vi "XY Graph Compute Sliced Mean & SDV Plots.vi"(8 "error in (no error)":errorcluster, 10 "Plot":cluster{"X Array":dbl[], "Y Array":dbl[]}, 11 "Slices Definition":T1={"Axis Start"=0.0, "Axis Stop"=0.0, "# Steps"=0, "Step Size"=1.0, "Step Definition"=enum."# Steps", "Upper Percentile"=1.0, "Lower Percentile"=1.0, "Min # Data Points/Slice"=1, "Output Abscissa Statistics Plots"=FALSE} {"Min # Data Points/Slice" min=0 max=100; "Lower Percentile" min=0.0 max=100.0; "Upper Percentile" min=0.0 max=100.0; "Step Size" min=1.0; "# Steps" min=1}) -> (0 "error out":errorcluster, 3 "Plots":cluster{"X Array":dbl[], "Y Array":dbl[]}[](array[cluster]))   [LabVIEW 2021, in "XY Graph Add-Ons.lvlib"]
uses:
  XY Graph Add-Ons.lvlib
  XY Graph Slides Mean & SDV Step Definition.ctl
  Arrays/Linear Ramp End Options.ctl
  49f03c9f-9bb8-4480-9460-08b8970c46f1.vi
  f2368cde-c411-4778-92ad-cdfa6392accb.vi
  ad4c9e8f-85ce-46f2-8889-cace00dc3fba.vi
  <userlib>/_OpenG.lib/array/array.llb/Sort 1D Array (DBL)__ogtk.vi
  <vilib>/Utility/error.llb/Error Cluster From Error Code.vi
  <vilib>/ErrorRing/Error Ring.xnode
  <vilib>/Comparison/Less/Less Functor/Less Functor.lvclass
  <vilib>/gmath/statdist.llb/st_Percentiles (array).vi
  <userlib>/_OpenG.lib/array/array.llb/Reorder 1D Array2 (DBL)__ogtk.vi
  Arrays/Arrays.lvlib
  <userlib>/_OpenG.lib/array/array.llb/openg_array.lvlib
  <vilib>/gmath/NI_Gmath.lvlib
  Comparison/Comparison.lvlib
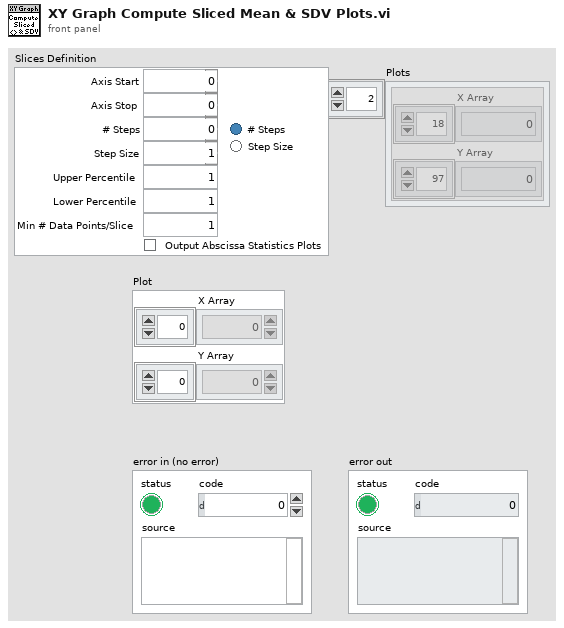
[diagram p1: front panel]
types:
  T1 = typedef "XY Graph Add-Ons.lvlib/XY Graph Slides Mean & SDV Step Definition.ctl" = cluster{"Axis Start":dbl, "Axis Stop":dbl, "# Steps":i32, "Step Size":dbl, "Step Definition":enum32{"# Steps", "Step Size"}, "Upper Percentile":dbl, "Lower Percentile":dbl, "Min # Data Points/Slice":i32, "Output Abscissa Statistics Plots":bool}
  T2 = typedef "Arrays.lvlib/Linear Ramp End Options.ctl" = enum16{"Include Min/Exclude Max", "Exclude Min/Include Max", "Include Both Ends", "Exclude Both Ends"}
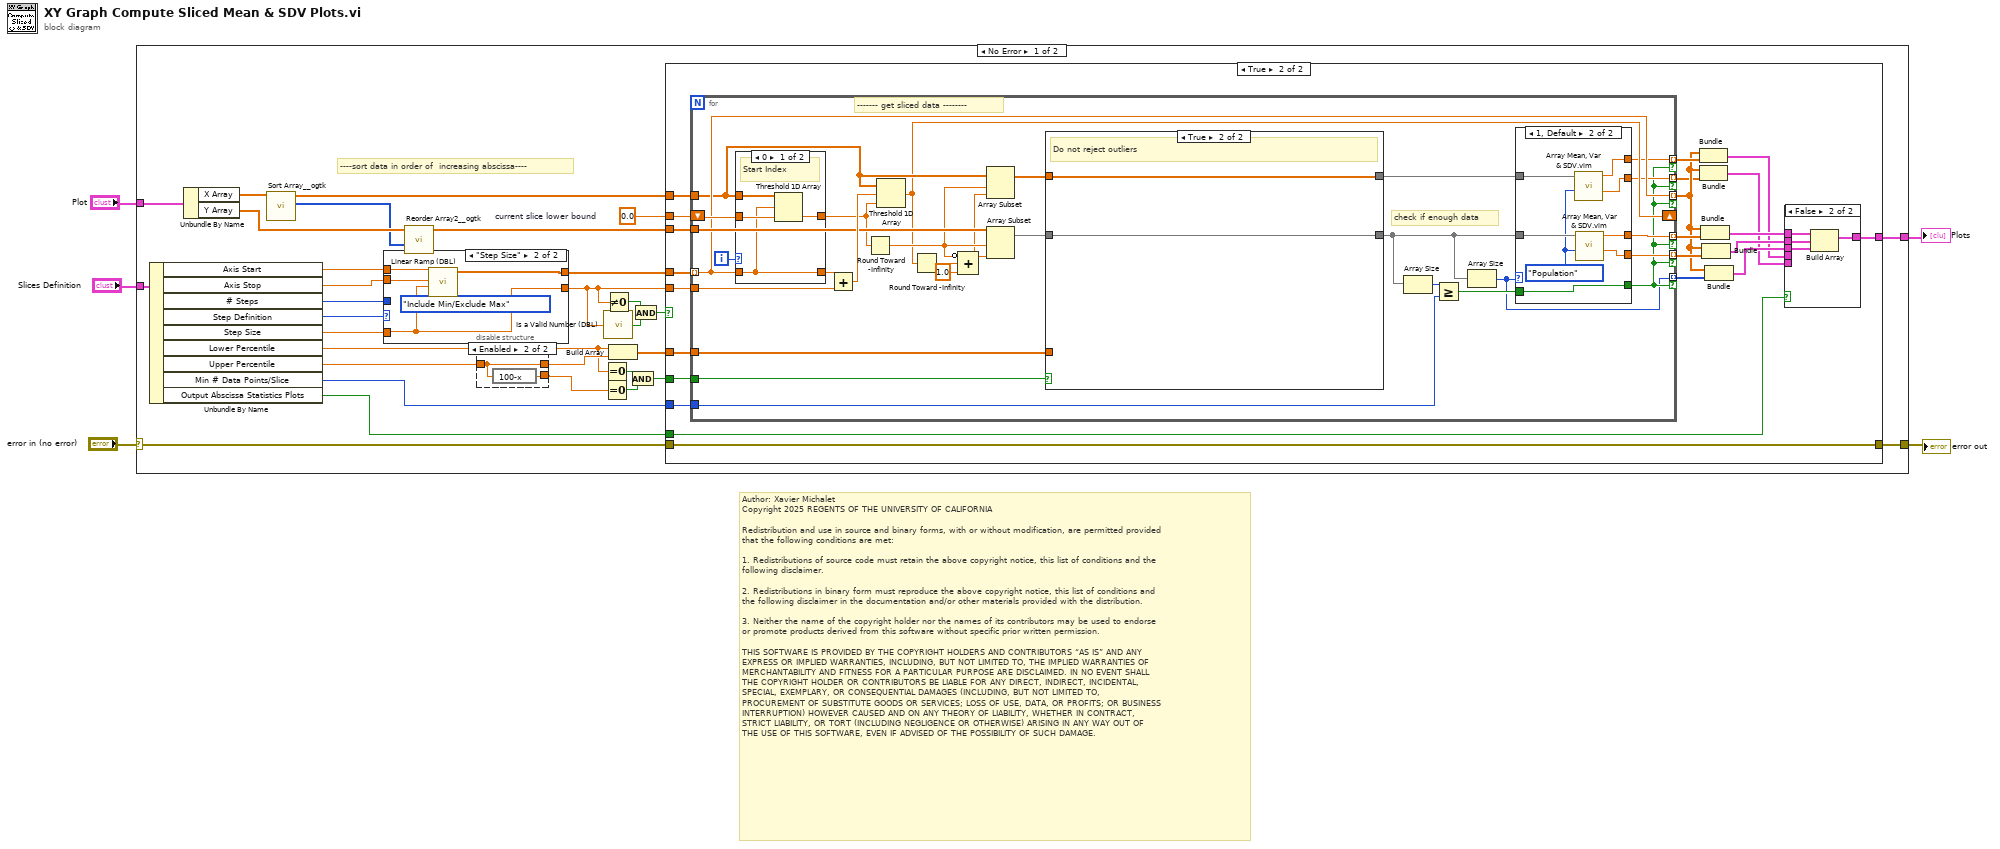
[diagram p0: block diagram]
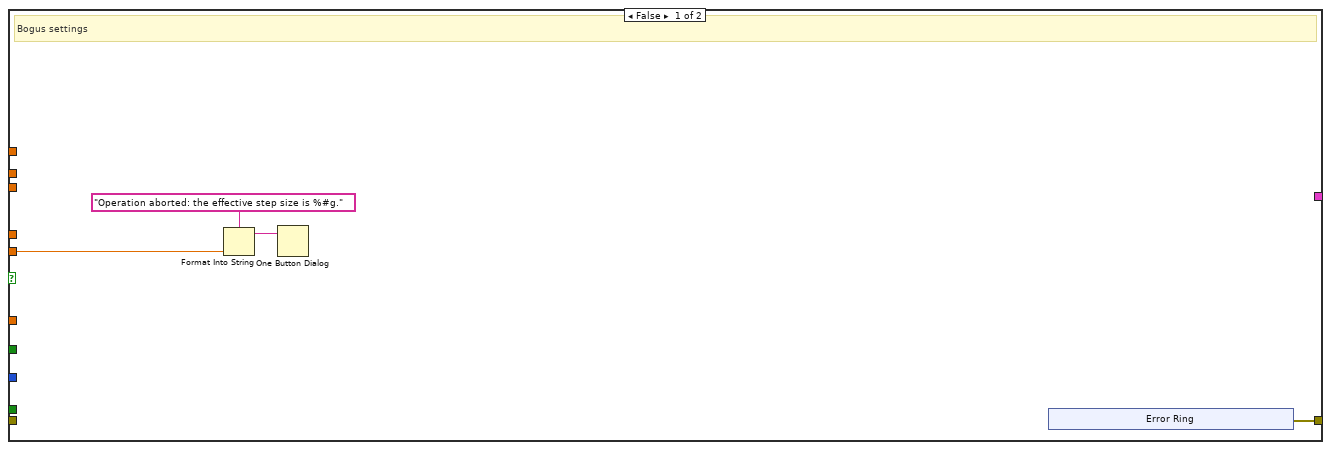
[diagram p2: hidden frame]
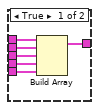
[diagram p3: hidden frame]
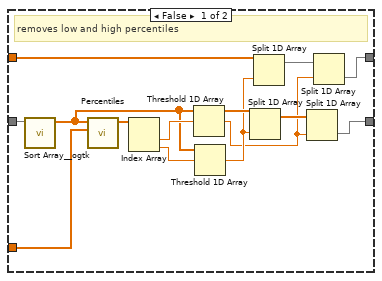
[diagram p4: hidden frame]
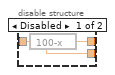
[diagram p7: hidden frame]
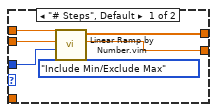
[diagram p8: hidden frame]
diagram:
  # "Author: Xavier Michalet\nCopyright 2025 REGENTS OF THE UNIVERSITY OF CALIFORNIA\n\nRedistribution and use in source and binary forms, with or without modification, are permitted provided\nthat the following conditions are met:\n\n1. Redistributions of source code must retain the above copyright notice, this list of conditions and the\nfollowing disclaimer.\n\n2. Redistributions in binary form must reproduce the above copyright notice, this list of conditions and\nthe following disclaimer in the documentation and/or other materials provided with the distribution.\n\n3. Neither the name of the copyright holder nor the names of its contributors may be used to endorse \nor promote products derived from this software without specific prior written permission.\n\nTHIS SOFTWARE IS PROVIDED BY THE COPYRIGHT HOLDERS AND CONTRIBUTORS “AS IS” AND ANY \nEXPRESS OR IMPLIED WARRANTIES, INCLUDING, BUT NOT LIMITED TO, THE IMPLIED WARRANTIES OF\nMERCHANTABILITY AND FITNESS FOR A PARTICULAR PURPOSE ARE DISCLAIMED. IN NO EVENT SHALL\nTHE COPYRIGHT HOLDER OR CONTRIBUTORS BE LIABLE FOR ANY DIRECT, INDIRECT, INCIDENTAL, \nSPECIAL, EXEMPLARY, OR CONSEQUENTIAL DAMAGES (INCLUDING, BUT NOT LIMITED TO, \nPROCUREMENT OF SUBSTITUTE GOODS OR SERVICES; LOSS OF USE, DATA, OR PROFITS; OR BUSINESS\nINTERRUPTION) HOWEVER CAUSED AND ON ANY THEORY OF LIABILITY, WHETHER IN CONTRACT, \nSTRICT LIABILITY, OR TORT (INCLUDING NEGLIGENCE OR OTHERWISE) ARISING IN ANY WAY OUT OF\nTHE USE OF THIS SOFTWARE, EVEN IF ADVISED OF THE POSSIBILITY OF SUCH DAMAGE."
  n1 = case shown="No Error" "error in (no error)" {
    selector: "error in (no error)" -> [w7 w150]
    tunnel: "Plot" -> [w36 _]
    tunnel: "Slices Definition" -> [w35 _]
    tunnel: [w25 _] -> w3
    tunnel: [w6 w150] -> w1
    frame No Error {
      w26 = 0.0  # current slice lower bound
      # "----sort data in order of  increasing abscissa----"
      n2 = Unbundle By Name(w35) -> ("Axis Start"=w34:dbl, "Axis Stop"=w33:dbl, "# Steps"=w32:i32, "Step Definition"=w24:enum32{"# Steps", "Step Size"}, "Step Size"=w23:dbl, "Lower Percentile"=w19:dbl, "Upper Percentile"=w14:dbl, "Min # Data Points/Slice"=w17:i32, "Output Abscissa Statistics Plots"=w12:bool)
      n3 = Unbundle By Name(w36) -> ("X Array"=w31:dbl[], "Y Array"=w30:dbl[])
      n4 = call-poly <userlib>:"Sort Array__ogtk.vi"("Array in"=w31) -> ("Sorted Pointers"=w29:i32[], "Sorted Array out"=w28:dbl[])  [unwired: 9 in]
      n5 = case shown="\"Step Size\"" w24 {
        tunnel: w34 -> [w144 w149]
        tunnel: w33 -> [w143 w148]
        tunnel: w32 -> [w142 _]
        tunnel: [w140 w145] -> w11
        tunnel: [w139 w146] -> w22
        tunnel: w23 -> [_ w145]
        frame "# Steps", Default {
          n6 = call "Linear Ramp by Number.vim"("Options"=Linear_Ramp_End_Options."Include Min/Exclude Max", "# Steps (1)"=w142, "End (1)"=w143, "Start (0)"=w144) -> ("Step Size"=w140:dbl, "Ramp"=w139:dbl[])  [unwired: 5 in, 1 out]
        }
        frame "Step Size" {
          n7 = call "Linear Ramp (DBL).vi"("Options"=Linear_Ramp_End_Options."Include Min/Exclude Max", "Delta"=w145, "Max"=w148, "Min"=w149) -> ("Ramp"=w146:dbl[])  [unwired: 6 in, 1 out]
        }
      }
      n8 = call-poly <userlib>:"Reorder Array2__ogtk.vi"("indices"=w29, "array"=w30) -> ("reordered array"=w27:dbl[])  [unwired: 9 in]
      n9 = disable-structure shown="Enabled" {
        disable-tunnel: [w136 w137] -> w20
        disable-tunnel: w14 -> [w135 w137]
        disable-tunnel: [w135 w138] -> w13
        frame Disabled {
          n10 = expression code="100-x"(w135) -> (w136:dbl)
        }
        frame Enabled {
          n11 = expression code="100-x"(w137) -> (w138:dbl)
        }
      }
      n12 = Equal To 0?(x=w19) -> (x = 0?=w18:bool)
      n13 = Equal To 0?(x=w13) -> (x = 0?=w16:bool)
      n14 = call "Is a Valid Number (DBL).vi"("Number"=w11) -> ("Valid Number?"=w9:bool)  [unwired: 8 in]
      n15 = Not Equal To 0?(x=w11) -> (x != 0?=w10:bool)
      n16 = Build Array(w19, w20) -> (w21:dbl[])
      n17 = And(x=w18, y=w16) -> (x .and. y?=w15:bool)
      n18 = And(x=w10, y=w9) -> (x .and. y?=w8:bool)
      n19 = case shown="True" w8 {
        tunnel: w28 -> [_ w66]
        tunnel: w27 -> [_ w65]
        tunnel: w26 -> [_ w64]
        tunnel: [_ w59] -> w25
        tunnel: w22 -> [_ w58]
        tunnel: w21 -> [_ w55]
        tunnel: w17 -> [_ w54]
        tunnel: w15 -> [_ w53]
        tunnel: w12 -> [_ w47]
        tunnel: w11 -> [w38 w46]
        tunnel: w7 -> [_ w45]
        tunnel: [w37 w45] -> w6
        frame False {
          # "Bogus settings"
          n20 = Format Into String(format string="Operation aborted: the effective step size is %#g.", w38) -> (resulting string=w40:string)  [unwired: 2 in, 1 out]
          n21 = One Button Dialog(message=w40) -> ()  [unwired: 1 in, 1 out]
          n22 = xnode "Error Ring"() -> ("error out"=w37:errorcluster)
        }
        frame True {
          n23 = for {
            tunnel: w58 -> [w91] mode=indexing
            tunnel: w66 -> [w86]
            tunnel: w65 -> [w100]
            shift-right: [w82] -> _
            shift-left: w64 -> [w104]
            tunnel: w46 -> [w102]
            tunnel: [w96] -> w63 mode=indexing if=w78
            tunnel: [w95] -> w62 mode=indexing if=w78
            tunnel: [w77] -> w57 mode=indexing if=w78
            tunnel: w55 -> [w94]
            tunnel: w54 -> [w92]
            tunnel: [w91] -> w51 mode=indexing if=w78
            tunnel: w53 -> [w87]
            tunnel: [w80] -> w52 mode=indexing if=w78
            tunnel: [w79] -> w50 mode=indexing if=w78
            i -> [w105]
            # "------- get sliced data --------"
            # "check if enough data"
            n24 = case shown="0" w105 {
              tunnel: w86 -> [w132 _]
              tunnel: w91 -> [w129 w134]
              tunnel: w104 -> [w131 w133]
              tunnel: [w130 w133] -> w99
              tunnel: [w129 w134] -> w103
              frame 0 {
                # "Start Index"
                n25 = Threshold 1D Array(1:w131, 2:w129, 3:w132) -> (0:w130:dbl)
              }
              frame 1, Default {
              }
            }
            n26 = Add(x=w103, y=w102) -> (x+y=w101:dbl)
            n27 = Round Toward -Infinity(1:w99) -> (0:w85:dbl)
            n28 = Threshold 1D Array(1:w99, 2:w101, 3:w86) -> (0:w82:dbl)
            n29 = Round Toward -Infinity(1:w82) -> (0:w98:dbl)
            n30 = Compound Arithmetic op=ADD(invert w85, w98, 1.0 ("value")) -> (w84:dbl)
            n31 = Array Subset(array=w86, index=w85, length=w84) -> (w83:dbl[])
            n32 = Array Subset(array=w100, index=w85, length=w84) -> (w88:dbl[])
            n33 = case shown="True" w87 {
              tunnel: w94 -> [w118 _]
              tunnel: [w116 w120] -> w93
              tunnel: w88 -> [w112 w120]
              tunnel: w83 -> [w110 w119]
              tunnel: [w107 w119] -> w81
              frame False {
                # "removes low and high percentiles"
                n34 = call-poly <userlib>:"Sort Array__ogtk.vi"("Array in"=w112) -> ("Sorted Array out"=w111:dbl[])  [unwired: 9 in, 1 out]
                n35 = call-poly <vilib>:"Percentiles.vi"("p array"=w118, "x array"=w111) -> ("percentiles"=w117:dbl[])  [unwired: 8 in, 1 out]
                n36 = Index Array(array=w117) -> (element #1=w115:dbl, element #2=w113:dbl)  [unwired: 2 in]
                n37 = Threshold 1D Array(2:w115, 3:w111) -> (0:w106:dbl)  [unwired: 1 in]
                n38 = Threshold 1D Array(2:w113, 3:w111) -> (0:w109:dbl)  [unwired: 1 in]
                n39 = Split 1D Array(array=w111, index=w109) -> (first subarray=w114:dbl[])  [unwired: 1 out]
                n40 = Split 1D Array(array=w110, index=w109) -> (first subarray=w108:dbl[])  [unwired: 1 out]
                n41 = Split 1D Array(array=w114, index=w106) -> (second subarray=w116:dbl[])  [unwired: 1 out]
                n42 = Split 1D Array(array=w108, index=w106) -> (second subarray=w107:dbl[])  [unwired: 1 out]
              }
              frame True {
                # "Do not reject outliers"
              }
            }
            n43 = Array Size(array=w93) -> (size(s)=w89:i32)
            n44 = Greater Or Equal?(x=w89, y=w92) -> (x >= y?=w90:bool)
            n45 = Array Size(array=w93) -> (size(s)=w77:i32)
            n46 = case shown="1, Default" w77 {
              tunnel: [_ w128] -> w96
              tunnel: [_ w127] -> w95
              tunnel: w93 -> [_ w126]
              tunnel: w90 -> [_ w125]
              tunnel: [_ w125] -> w78
              tunnel: w81 -> [_ w124]
              tunnel: [_ w122] -> w80
              tunnel: [_ w121] -> w79
              frame 0 {
              }
              frame 1, Default {
                w123 = enum16{"Sample", "Population"}."Population" ("Weighting (Sample)")
                n47 = call "Array Mean, Var & SDV.vim"("Weighting (Sample)"=w123, "Array"=w124) -> ("Array SDV"=w121:dbl, "Array Mean"=w122:dbl)  [unwired: 6 in, 2 out]
                n48 = call "Array Mean, Var & SDV.vim"("Weighting (Sample)"=w123, "Array"=w126) -> ("Array SDV"=w127:dbl, "Array Mean"=w128:dbl)  [unwired: 6 in, 2 out]
              }
            }
          }
          n49 = Bundle(w51, w52) -> (w49:cluster{dbl[], dbl[]})  [unwired: 1 in]
          n50 = Bundle(w51, w50) -> (w48:cluster{dbl[], dbl[]})  [unwired: 1 in]
          n51 = Bundle(w51, w63) -> (w61:cluster{dbl[], dbl[]})  [unwired: 1 in]
          n52 = Bundle(w51, w62) -> (w60:cluster{dbl[], dbl[]})  [unwired: 1 in]
          n53 = Bundle(w51, w57) -> (w56:cluster{dbl[], i32[]})  [unwired: 1 in]
          n54 = case shown="False" w47 {
            tunnel: w61 -> [w72 w76]
            tunnel: w60 -> [w71 w75]
            tunnel: [w70 w74] -> w59
            tunnel: w56 -> [w69 w73]
            tunnel: w49 -> [w68 _]
            tunnel: w48 -> [w67 _]
            frame True {
              n55 = Build Array(w72, w71, w69, w68, w67) -> (w70:cluster{dbl[], dbl[]}[])
            }
            frame False {
              n56 = Build Array(w76, w75, w73) -> (w74:cluster{dbl[], dbl[]}[])
            }
          }
        }
      }
    }
    frame Error {
    }
  }
  "error out" <- w1
  "Plots" <- w3
